vi "Get Currents & Ranges.vi"(0 "TCS.lvclass in":refnum<class "TCS.lvclass">, 5 "error in (no error)":errorcluster) -> (14 "TCS.lvclass out":refnum<class "TCS.lvclass">, 15 "I0":cluster{"Value":dbl, "Range":dbl}, 16 "I1":cluster{"Value":dbl, "Range":dbl}, 17 "I2":cluster{"Value":dbl, "Range":dbl}, 18 "I3":cluster{"Value":dbl, "Range":dbl}, 19 "error out":errorcluster)   [LabVIEW 2016, in "TCS.lvclass"]
uses:
  Lib.llb/TCS.lvclass
  Lib.llb/CS.lvclass
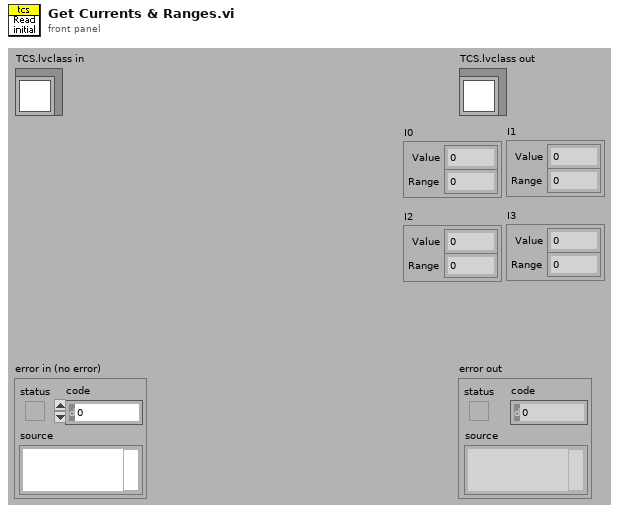
[diagram p1: front panel]
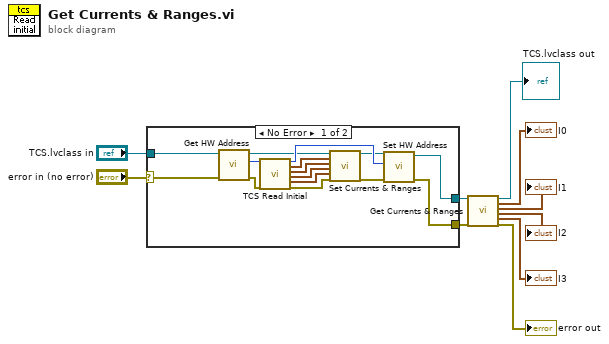
[diagram p0: block diagram]
diagram:
  n1 = case shown="No Error" "error in (no error)" {
    selector: "error in (no error)" -> [w21 w27]
    tunnel: [w20 w27] -> w3
    tunnel: "TCS.lvclass in" -> [w24 w26]
    tunnel: [w23 w26] -> w1
    frame No Error {
      n2 = call-dynamic "Get HW Address.vi"("error in (no error)"=w21, "CS.lvclass in"=w24) -> ("error out"=w22:errorcluster, "HW Address"=w25:i32, "CS.lvclass out"=w17:refnum<class "TCS.lvclass">)  [unwired: 7 in]
      n3 = call "TCS Read Initial.vi"("port number in"=w25, "error in"=w22) -> ("port number out"=w19:u8, "CS0"=w16:cluster{"Value":sgl, "Range":u8}, "CS1"=w15:cluster{"Value":sgl, "Range":u8}, "CS2"=w14:cluster{"Value":sgl, "Range":u8}, "CS3"=w13:cluster{"Value":sgl, "Range":u8}, "error out"=w12:errorcluster)  [unwired: 12 in]
      n4 = call-dynamic "Set Currents & Ranges.vi"("CS.lvclass in"=w17, "I0"=w16, "I1"=w15, "I2"=w14, "I3"=w13, "error in (no error)"=w12) -> ("CS.lvclass out"=w18:refnum<class "TCS.lvclass">, "error out"=w11:errorcluster)  [unwired: 12 in]
      n5 = call-dynamic "Set HW Address.vi"("error in (no error)"=w11, "HW Address"=w19, "CS.lvclass in"=w18) -> ("error out"=w20:errorcluster, "CS.lvclass out"=w23:refnum<class "TCS.lvclass">)  [unwired: 7 in]
    }
    frame Error {
    }
  }
  n6 = call-parent "Get Currents & Ranges.vi"("CS.lvclass in"=w1, "error in (no error)"=w3) -> ("CS.lvclass out"=→"TCS.lvclass out":refnum<class "TCS.lvclass">, "I0"=→"I0":cluster{"Value":dbl, "Range":dbl}, "I1"=→"I1":cluster{"Value":dbl, "Range":dbl}, "I2"=→"I2":cluster{"Value":dbl, "Range":dbl}, "I3"=→"I3":cluster{"Value":dbl, "Range":dbl}, "error out"=→"error out":errorcluster)  [unwired: 12 in]
